vi "create-path-trajectory.vi"() -> ()   [LabVIEW 2019]
uses:
  <vilib>/Rock Robotics/WPI/ThirdParty/JAS_Junk/TrajLib/TypeDef/TRANSLATION2D.ctl
  <vilib>/Rock Robotics/WPI/ThirdParty/JAS_Junk/TrajLib/Trajectory_Library.lvlib
panel:
  in  "Position 4":T1={"X"=1.0, "Y"=4.0} {"Y" format="%14.3f"; "X" format="%14.3f"}
  in  "Position 3":T1={"X"=1.0, "Y"=3.0} {"Y" format="%14.3f"; "X" format="%14.3f"}
  in  "Position 2":T1={"X"=1.0, "Y"=2.0} {"Y" format="%14.3f"; "X" format="%14.3f"}
  in  "Position 1":T1={"X"=1.0, "Y"=1.0} {"Y" format="%14.3f"; "X" format="%14.3f"}
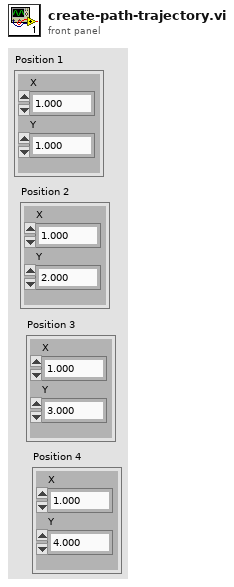
[diagram p1: front panel]
types:
  T1 = typedef "Trajectory_Library.lvlib/TRANSLATION2D.ctl" = cluster{"X":dbl, "Y":dbl}
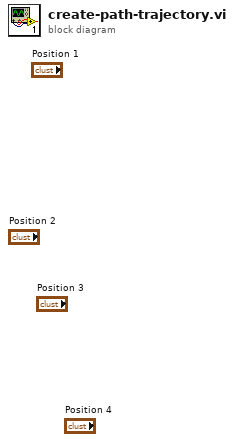
[diagram p0: block diagram]
diagram:
